vi "Delay.vi"(11 "address":refnum<class "Generic Network Address.lvclass">) -> (3 "address out":refnum<class "Generic Network Address.lvclass">)   [LabVIEW 2020, in "NI_WFCN.lvlib" / "Generic Network Address.lvclass"]
doc: "Wait a little while for the network configuration to possibly change."
uses:
  <vilib>/net/WFCN/Addressing/Generic Network Address/Generic Network Address.lvclass
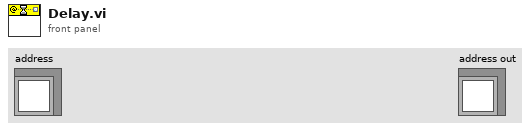
[diagram p1: front panel]
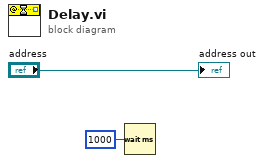
[diagram p0: block diagram]
diagram:
  n1 = Wait (ms)(milliseconds to wait=u32 1000) -> ()  [unwired: 1 out]
  "address out" <- "address"
